vi "Timer Logic.vi"(3 "Reset":bool, 4 "Delay":u32, 5 "Timer In":u32) -> (0 "End Trigger":bool, 1 "Start Trigger":bool, 2 "Timer Out":u32)   [LabVIEW 2012, in "femtoRoboLib.lvlib"]
uses:
  femtoRoboLib.lvlib
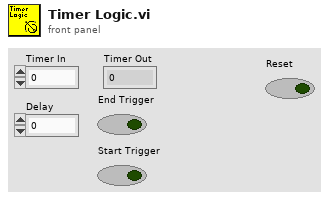
[diagram p1: front panel]
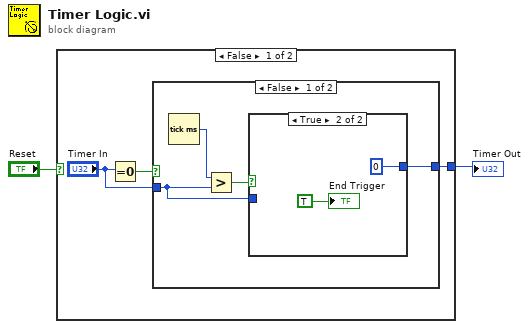
[diagram p0: block diagram]
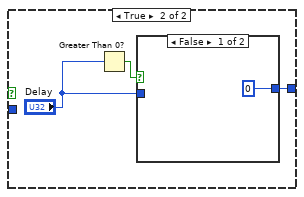
[diagram p3: hidden frame]
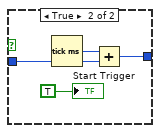
[diagram p4: hidden frame]
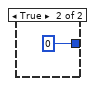
[diagram p5: hidden frame]
diagram:
  n1 = case shown="False" "Reset" {
    tunnel: [w4 u32 0 ("Timer In")] -> w2
    frame False {
      n2 = Equal To 0?(x="Timer In") -> (x = 0?=w5:bool)
      n3 = case shown="False" w5 {
        tunnel: [w6 w15] -> w4
        tunnel: "Timer In" -> [w7 _]
        frame False {
          n4 = Tick Count (ms)() -> (millisecond timer value=w8:u32)
          n5 = Greater?(x=w8, y=w7) -> (0:w9:bool)
          n6 = case shown="True" w9 {
            tunnel: w7 -> [w10 _]
            tunnel: [w10 u32 0 ("Timer In")] -> w6
            frame False {
            }
            frame True {
              "End Trigger" <- TRUE ("Trigger")
            }
          }
        }
        frame True {
          n7 = Greater Than 0?(x="Delay") -> (x > 0?=w14:bool)
          n8 = case shown="False" w14 {
            tunnel: "Delay" -> [_ w19]
            tunnel: [u32 0 w18] -> w15
            frame False {
            }
            frame True {
              n9 = Tick Count (ms)() -> (millisecond timer value=w20:u32)
              n10 = Add(x=w20, y=w19) -> (x+y=w18:u32)
              "Start Trigger" <- TRUE ("Start Trigger")
            }
          }
        }
      }
    }
    frame True {
    }
  }
  "Timer Out" <- w2
